vi "alpha_0.2.vi"() -> ()   [LabVIEW 2018]
panel:
  in  "Timer (ms)":dbl
  in  "Switch":bool
  out "RED":bool
  out "YELLOW":bool
  out "GREEN":bool
  in  "?":bool
  in  "Emergency":bool
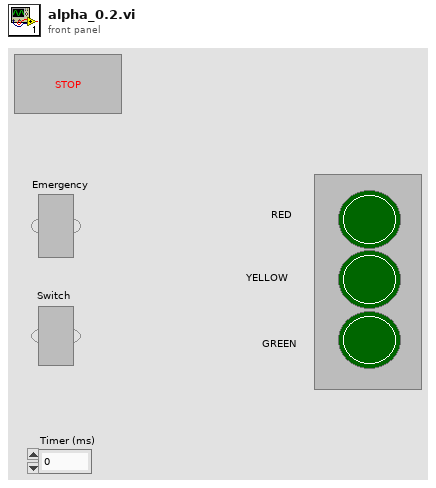
[diagram p1: front panel]
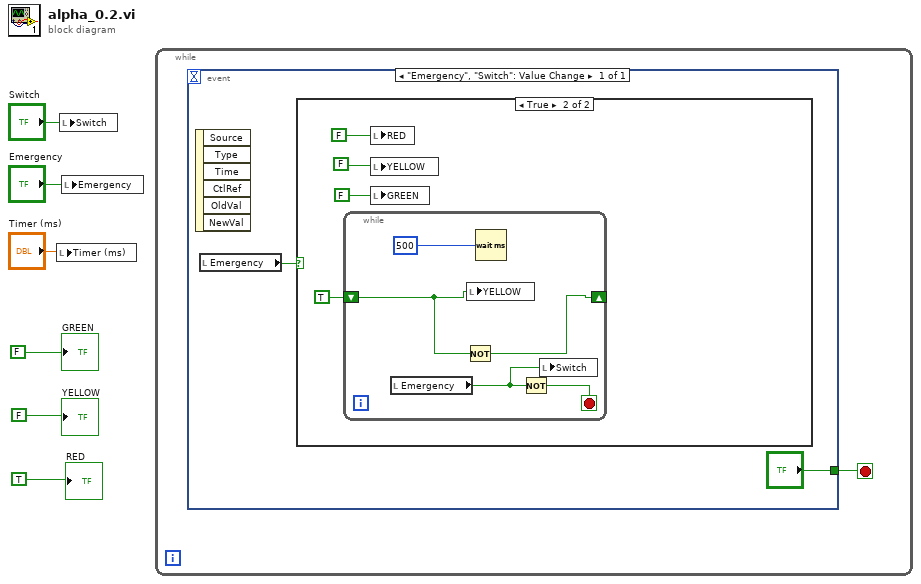
[diagram p0: block diagram]
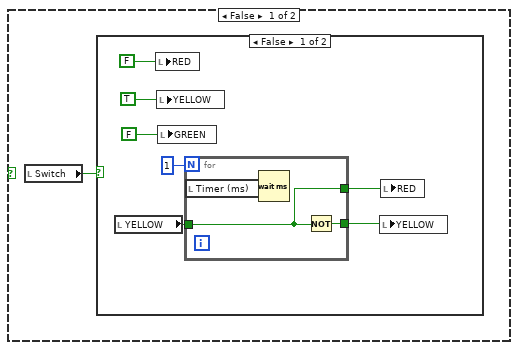
[diagram p2: hidden frame]
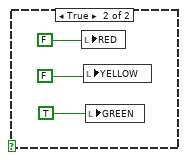
[diagram p3: hidden frame]
diagram:
  n1 = local write "Timer (ms)"("Timer (ms)") -> ()
  n2 = local write "Switch"("Switch") -> ()
  n3 = local write "Emergency"("Emergency") -> ()
  n4 = while {
    stop <- w7 stop-if-true
    n5 = event shown="[0] \"Emergency\", \"Switch\": Value Change" {
      selector: _ -> [_]
      dyn-events: _ -> [_]
      timeout: _ -> [_]
      tunnel: ["?"] -> w7
      event "Emergency", "Switch": Value Change {
        n6 = event-data() -> ()  [unwired: 1 in, 6 out]
        n7 = local read "Emergency"() -> (w9:bool)
        n8 = case shown="True" w9 {
          frame False {
            n9 = local read "Switch"() -> (w10:bool)
            n10 = case shown="False" w10 {
              frame False {
                n11 = local read "YELLOW"() -> (w14:bool)
                n12 = local write "RED"(FALSE) -> ()
                n13 = local write "YELLOW"(TRUE) -> ()
                n14 = local write "GREEN"(FALSE) -> ()
                n15 = for {
                  N: 1 -> [_]
                  tunnel: w14 -> [w19]
                  tunnel: [w20] -> w12
                  tunnel: [w19] -> w11
                  n16 = local read "Timer (ms)"() -> (w18:dbl)
                  n17 = Wait (ms)(milliseconds to wait=w18) -> ()  [unwired: 1 out]
                  n18 = Not(x=w19) -> (.not. x?=w20:bool)
                }
                n19 = local write "YELLOW"(w12) -> ()
                n20 = local write "RED"(w11) -> ()
              }
              frame True {
                n21 = local write "RED"(FALSE) -> ()
                n22 = local write "YELLOW"(FALSE) -> ()
                n23 = local write "GREEN"(TRUE) -> ()
              }
            }
          }
          frame True {
            n24 = while {
              shift-right: [w31] -> _
              shift-left: TRUE -> [w32]
              stop <- w29 stop-if-true
              n25 = local read "Emergency"() -> (w28:bool)
              n26 = Not(x=w32) -> (.not. x?=w31:bool)
              n27 = local write "YELLOW"(w32) -> ()
              n28 = Wait (ms)(milliseconds to wait=500) -> ()  [unwired: 1 out]
              n29 = Not(x=w28) -> (.not. x?=w29:bool)
              n30 = local write "Switch"(w28) -> ()
            }
            n31 = local write "RED"(FALSE) -> ()
            n32 = local write "YELLOW"(FALSE) -> ()
            n33 = local write "GREEN"(FALSE) -> ()
          }
        }
      }
    }
  }
  "GREEN" <- FALSE
  "YELLOW" <- FALSE
  "RED" <- TRUE
